vi "Create.vi"(8 "error in (no error)":errorcluster) -> (0 "error out":errorcluster, 3 "Event Registration Refnum":refnum<event-registration>)   [LabVIEW 2020, in "WebServiceImporter.lvlib" / "Main Panel.lvlib" / "Events.lvlib"]
uses:
  <vilib>/Platform/WebService/Main Panel/Events/Events.lvlib
  <vilib>/Platform/WebService/Main Panel/Events/Data Type/Page.ctl
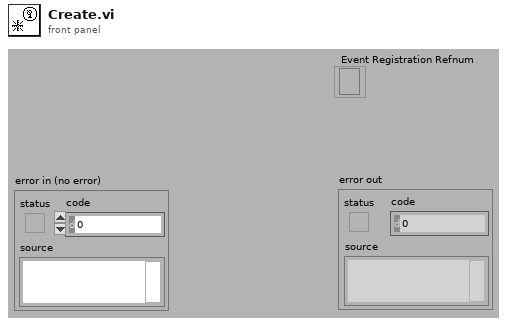
[diagram p1: front panel]
types:
  T1 = typedef "WebServiceImporter.lvlib/Main Panel.lvlib/Events.lvlib/Page.ctl" = enum16{"Input WSDL", "Input Authentication", "Input Info", "Select Methods", "Preview", "Progress", "Finish"}
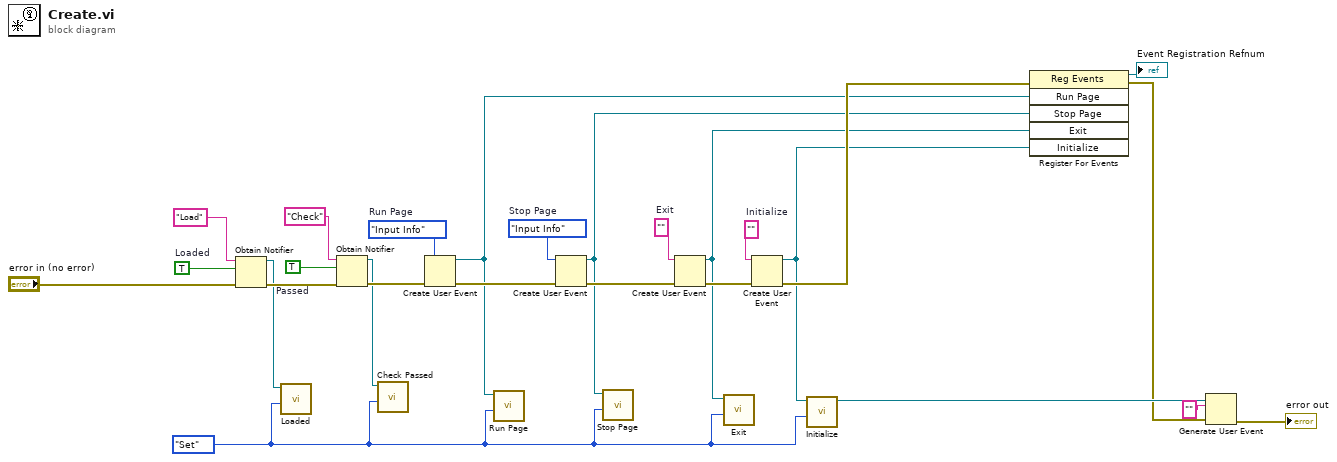
[diagram p0: block diagram]
diagram:
  w5 = TRUE  # Passed
  w6 = TRUE  # Loaded
  w2 = enum16{"Get", "Set"}."Set" ("Operation")
  w27 = Page."Input Info"  # Run Page
  w25 = Page."Input Info"  # Stop Page
  w23 = ""  # Exit
  w21 = ""  # Initialize
  n1 = Obtain Notifier(name (unnamed)="Load", notification data type=w6, error in (no error)="error in (no error)") -> (notifier out=w4:refnum<notifier>, error out=w10:errorcluster)  [unwired: 1 in, 1 out]
  n2 = call <vilib>:"Loaded.vi"("Operation"=w2, "notifier"=w4) -> ()  [unwired: 9 in, 1 out]
  n3 = Obtain Notifier(name (unnamed)="Check", notification data type=w5, error in (no error)=w10) -> (notifier out=w3:refnum<notifier>, error out=w9:errorcluster)  [unwired: 1 in, 1 out]
  n4 = call <vilib>:"Check Passed.vi"("Operation"=w2, "notifier"=w3) -> ()  [unwired: 8 in, 2 out]
  n5 = Create User Event(user event datatype=w27, error in=w9) -> (user event=w13:refnum<user-event>, error out=w26:errorcluster)
  n6 = call <vilib>:"Run Page.vi"("Operation"=w2, "user event"=w13) -> ()  [unwired: 9 in, 1 out]
  n7 = Create User Event(user event datatype=w25, error in=w26) -> (user event=w12:refnum<user-event>, error out=w24:errorcluster)
  n8 = call <vilib>:"Stop Page.vi"("Operation"=w2, "user event"=w12) -> ()  [unwired: 9 in, 1 out]
  n9 = Create User Event(user event datatype=w23, error in=w24) -> (user event=w16:refnum<user-event>, error out=w22:errorcluster)
  n10 = call <vilib>:"Exit.vi"("Operation"=w2, "user event"=w16) -> ()  [unwired: 9 in, 1 out]
  n11 = Create User Event(user event datatype=w21, error in=w22) -> (user event=w18:refnum<user-event>, error out=w20:errorcluster)
  n12 = call <vilib>:"Initialize.vi"("Operation"=w2, "user event"=w18) -> ("user event out"=w17:refnum<user-event>)  [unwired: 9 in]
  n13 = register-events(error in=w20, w13, w12, w16, w18) -> (reference out=→"Event Registration Refnum":refnum<event-registration>, error out=w15:errorcluster)  [unwired: 1 in]
  n14 = Generate User Event(user event=w17, event data cluster="" ("event data"), error in=w15) -> (error out=→"error out":errorcluster)  [unwired: 1 in, 1 out]
